vi "RescalePixelToAODFrequency.vi"(4 "FlipY":bool, 6 "FlipX":bool, 10 "Pixels":i32[](array[numeric]), 11 "?":T1={"Calibration Input"=[], "CalibrationResults"={"Center in Pixels"=[374.0120339529387, 375.46592887074246], "Angle"=0.022945275255000355, "Pixels/MHz X"=0.0, "Pixels/MHz Y"=0.0}, "Highlight"=[], "Running Script"=refnum}) -> (3 "Array":dbl[](array[numeric]))   [LabVIEW 2017]
uses:
  ExperimentVariables.ctl
  <vilib>/Analysis/coordinate.llb/2D Cartesian Coordinate Rotation (Scalar).vi
  <vilib>/Analysis/NI_AALPro.lvlib
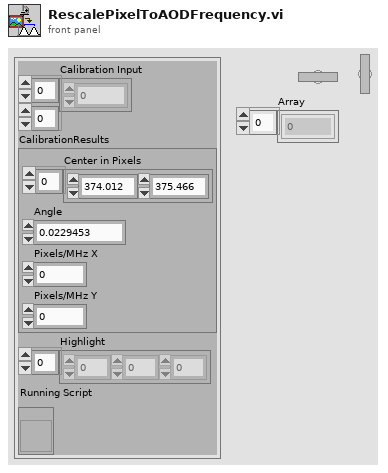
[diagram p1: front panel]
types:
  T1 = typedef "ExperimentVariables.ctl" = cluster{"Calibration Input":i32[][], "CalibrationResults":cluster{"Center in Pixels":dbl[], "Angle":dbl, "Pixels/MHz X":dbl, "Pixels/MHz Y":dbl}, "Highlight":i32[], "Running Script":refnum<vi>}
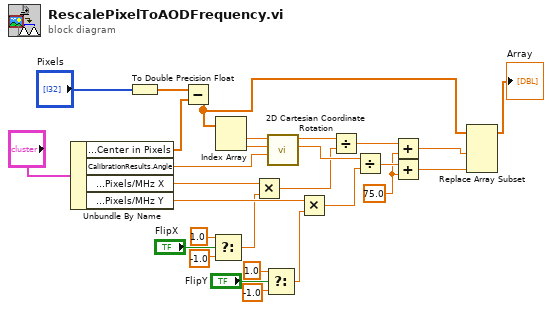
[diagram p0: block diagram]
diagram:
  w16 = 75.0 ("y")
  n1 = Unbundle By Name("?") -> ("CalibrationResults.Center in Pixels"=w25:dbl[], "CalibrationResults.Angle"=w22:dbl, "CalibrationResults.Pixels/MHz X"=w9:dbl, "CalibrationResults.Pixels/MHz Y"=w12:dbl)
  n2 = To Double Precision Float(number="Pixels") -> (double precision float=w27:dbl[])
  n3 = Subtract(x=w27, y=w25) -> (x-y=w19:dbl[])
  n4 = Select(t=1.0, s="FlipX", f=-1.0 ("t")) -> (s? t:f=w2:dbl)
  n5 = Index Array(array=w19) -> (element #1=w24:dbl, element #2=w23:dbl)  [unwired: 2 in]
  n6 = Multiply(x=w9, y=w2) -> (x*y=w10:dbl)
  n7 = Select(t=1.0, s="FlipY", f=-1.0 ("t")) -> (s? t:f=w8:dbl)
  n8 = call-poly <vilib>:"2D Cartesian Coordinate Rotation.vi"("theta"=w22, "y"=w23, "x"=w24) -> ("y out"=w20:dbl, "x out"=w21:dbl)  [unwired: 6 in, 1 out]
  n9 = Multiply(x=w12, y=w8) -> (x*y=w11:dbl)
  n10 = Divide(x=w21, y=w10) -> (x/y=w17:dbl)
  n11 = Divide(x=w20, y=w11) -> (x/y=w18:dbl)
  n12 = Add(x=w17, y=w16) -> (x+y=w13:dbl)
  n13 = Add(x=w18, y=w16) -> (x+y=w14:dbl)
  n14 = Replace Array Subset(array=w19, new element #1=w13, new element #2=w14) -> (→"Array":dbl[])  [unwired: 2 in]
